vi "LVClass_ModalCoef ctor FromData.vi"(0 "ModalCoef (const)":refnum<class "ModalCoef.lvclass">, 1 "Pupil":refnum<class "Pupil.lvclass">, 5 "TypePhase":T1, 7 "coef":sgl[](array[numeric]), 9 "polyindex":i32[](array[numeric]), 11 "error in (no error)":errorcluster) -> (3 "Pupil (dup)":refnum<class "Pupil.lvclass">, 4 "ModalCoef (new)":refnum<class "ModalCoef.lvclass">, 15 "error out":errorcluster)   [LabVIEW 2020, in "ModalCoef.lvclass"]
doc: "ModalCoef constructor from reconstruction informations.\n\n--------------------------------------------------------------------------------\n\n<B>ModalCoefIn </B> : Constant Pointer to ModalCoef object.\n<B>ModalCoefOut </B> : Constant Pointer to ModalCoef object.\n<B>TypePhase </B> : TypePhase Phase mode reconstruction.\n<B>polyindex </B> : Array of modal coefficient indices.\n<B>coef </B> : Array of modal coefficient values.\n<B>pupil </B> : pupil object.\n<B>size </B> : Size of modal coefficient array.\n<B>ErrorIn </B> : Error\n<B>ErrorOut </B> : Error\n\n--------------------------------------------------------------------------------"
uses:
  ModalCoef.lvclass
  WavefrontModalReconstructionType.ctl
  Pupil.lvclass
  Handle creation.ctl
  ModalCoef.lvclass/ModalCoef.ctl
  LVClass_Pupil Read Pupil.vi
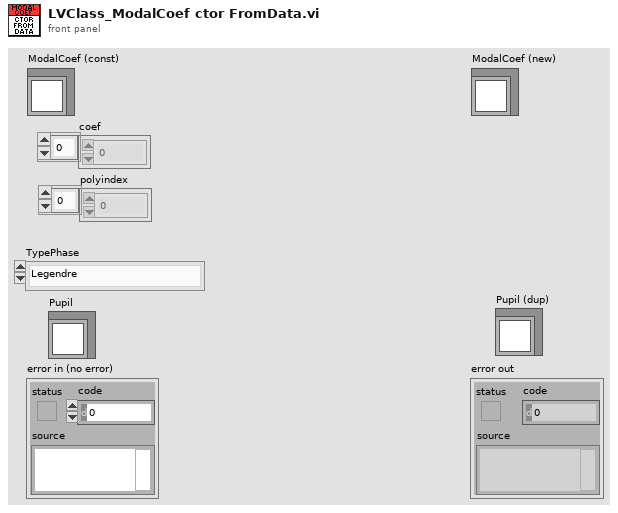
[diagram p1: front panel]
types:
  T1 = typedef "WavefrontModalReconstructionType.ctl" = enum16{"Legendre", "Zernike"}
  T2 = typedef "Handle creation.ctl" = enum16{"By ctor", "By write function"}
  T3 = typedef "ClassID.ctl" = i64
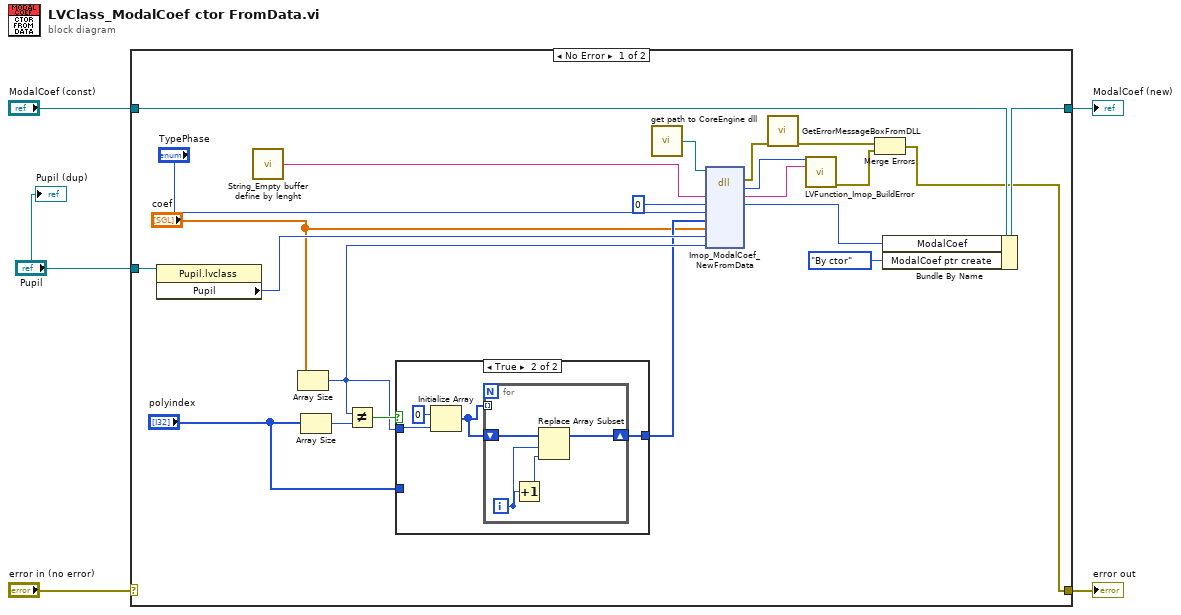
[diagram p0: block diagram]
diagram:
  n1 = case shown="No Error" "error in (no error)" {
    selector: "error in (no error)" -> [_ w38]
    tunnel: [w6 w38] -> w4
    tunnel: [w18 w37] -> w2
    tunnel: "ModalCoef (const)" -> [w19 w37]
    tunnel: "Pupil" -> [w17 _]
    frame No Error {
      n2 = property class="Pupil.lvclass"(reference=w17) -> ("Pupil"=w16:T3)  [unwired: 1 in, 2 out]
      n3 = call "String_Empty buffer define by lenght.vi"() -> ("Empty buffer"=w27:string)  [unwired: 1 in]
      n4 = Array Size(array="coef") -> (size(s)=w12:i32)
      n5 = Array Size(array="polyindex") -> (size(s)=w14:i32)
      n6 = Not Equal?(x=w12, y=w14) -> (x != y?=w13:bool)
      n7 = case shown="True" w13 {
        tunnel: w12 -> [_ w30]
        tunnel: "polyindex" -> [w28 _]
        tunnel: [w28 w29] -> w10
        frame False {
        }
        frame True {
          n8 = Initialize Array(u32 0, w30) -> (w31:u32[])
          n9 = for {
            shift-right: [w33] -> w29
            shift-left: w31 -> [w34]
            tunnel: w31 -> [_] mode=indexing
            i -> [w35]
            n10 = Increment(x=w35) -> (x+1=w36:i32)
            n11 = Replace Array Subset(array=w34, new element=w36, index=w35) -> (w33:u32[])
          }
        }
      }
      n12 = call "get path to CoreEngine dll.vi"() -> ("path to wavekit library"=w24:path)  [unwired: 14 in, 1 out]
      n13 = dll-call lib="D:/soft/HASO_v3/SVN_trunk/ImOpCoreEngine4_LV2011/DLLs/c_interface_vc100.dll" fn="Imop_ModalCoef_NewFromData"(path in=w24, "message"=w27, "ModalCoef"=0 ("Pupil"), "TypePhase"="TypePhase", "polyindex"=w10, "coef"="coef", "pupil"=w16, "size"=w12) -> (error out=w23:errorcluster, "return type"=w25:i32, "message"=w26:string, "ModalCoef"=w21:i64)  [unwired: 7 in, 1 out]
      n14 = call "GetErrorMessageBoxFromDLL.vi"("error IN"=w23) -> ("error OUT"=w8:errorcluster)  [unwired: 10 in]
      n15 = call "LVFunction_Imop_BuildError.vi"("code"=w25, "String to Prepend to source (\"\")"=w26) -> ("error out"=w7:errorcluster)  [unwired: 13 in]
      n16 = Merge Errors(w8, w7) -> (w6:errorcluster)
      n17 = Bundle By Name(cluster=w19, "ModalCoef"=w21, "ModalCoef ptr create"=Handle_creation."By ctor" ("Pupil ptr create")) -> (w18:refnum<class "ModalCoef.lvclass">)
    }
    frame Error {
    }
  }
  "error out" <- w4
  "ModalCoef (new)" <- w2
  "Pupil (dup)" <- "Pupil"
